vi "New SenseHat.Joystick.vi"(8 "error in (no error)":errorcluster, 11 "MainI2CDevice":refnum<class "mainI2CDevice.lvclass">) -> (0 "error out":errorcluster, 3 "senseHatJoystick out":refnum<class "RPI.SenseHat.Joystick.lvclass">)   [LabVIEW 2020, in "RPI.SenseHat.Joystick.lvlib" / "RPI.SenseHat.Joystick.lvclass"]
uses:
  RPI.SenseHat.Joystick.lvclass
  TypeDefs/Key State.ctl
  RPI.SenseHat.Joystick.lvlib
  RPI/Classes/mainI2CDevice/mainI2CDevice.lvclass
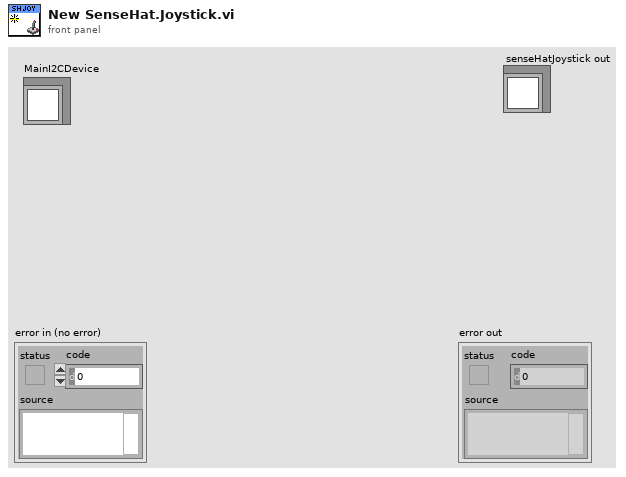
[diagram p1: front panel]
types:
  T1 = typedef "RPI.SenseHat.Joystick.lvlib/Key State.ctl" = enum16{"Released", "Pressing", "Pressed", "Releasing"}
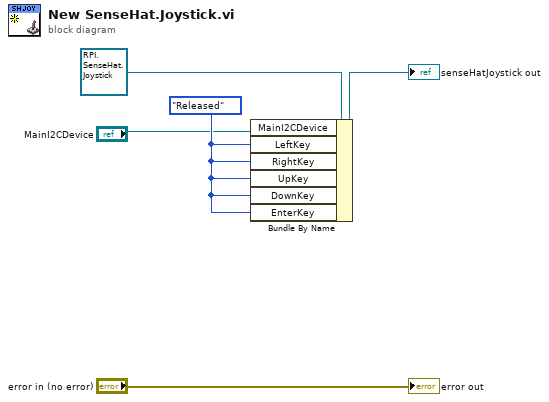
[diagram p0: block diagram]
diagram:
  w2 = Key_State."Released" ("DownKey")
  n1 = Bundle By Name(cluster=refnum<class "RPI.SenseHat.Joystick.lvclass"> refnum ("senseHatJoystick in"), "MainI2CDevice"="MainI2CDevice", "LeftKey"=w2, "RightKey"=w2, "UpKey"=w2, "DownKey"=w2, "EnterKey"=w2) -> (→"senseHatJoystick out":refnum<class "RPI.SenseHat.Joystick.lvclass">)
  "error out" <- "error in (no error)"
